vi "Run Bfr Rx - Flag Rollover.vi"(7 "Offset in":u64, 8 "error in (no error)":errorcluster, 10 "Rollover?":bool, 11 "Data Buffer in":u64 format="%016x") -> (0 "error out":errorcluster)   [LabVIEW 2016, in "UDP-Custom-Device Engine.lvlib"]
uses:
  UDP-Custom-Device Engine.lvlib
  <vilib>/NI Veristand/VeriStand Data/Library/Pointer Operations/Pointer.Write (I32).vi
  <vilib>/NI Veristand/VeriStand Data/Library/VeriStand Data.lvlib
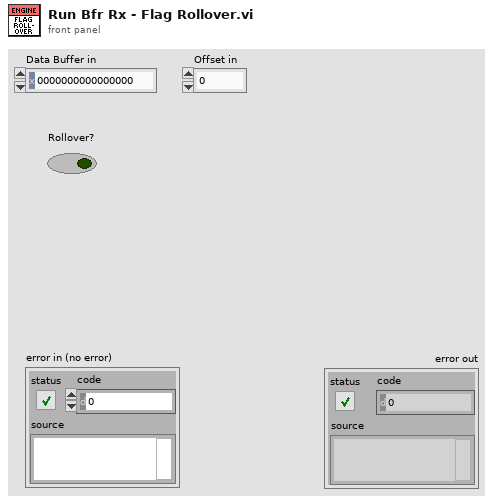
[diagram p1: front panel]
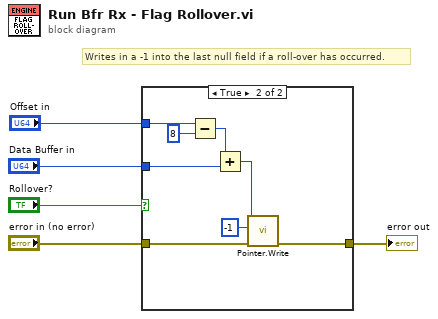
[diagram p0: block diagram]
diagram:
  # "Writes in a -1 into the last null field if a roll-over has occurred."
  n1 = case shown="True" "Rollover?" {
    tunnel: "error in (no error)" -> [w6 w14]
    tunnel: [w6 w13] -> w4
    tunnel: "Data Buffer in" -> [_ w8]
    tunnel: "Offset in" -> [_ w11]
    frame False {
    }
    frame True {
      n2 = Subtract(x=w11, y=u64 8) -> (x-y=w10:u64)
      n3 = Add(x=w10, y=w8) -> (x+y=w7:u64)
      n4 = call-poly <vilib>:"Pointer.Write.vi"("error in (no error)"=w14, "value"=-1, "pointer in"=w7) -> ("error out"=w13:errorcluster)  [unwired: 6 in, 2 out]
    }
  }
  "error out" <- w4
